vi "DT_Divide.vi"(10 "min subset size":i32=4, 11 "Points In":cluster{"x":dbl, "y":dbl, "index":i32}[](array[cluster])) -> (2 "Subset":cluster{"start idx":i32, "length":i32}[](array[cluster]), 3 "Points Out":cluster{"x":dbl, "y":dbl, "index":i32}[](array[cluster]))   [LabVIEW 2020, in "NI_AAL_Geometry.lvlib"]
uses:
  <vilib>/Analysis/NI_AAL_Geometry.lvlib
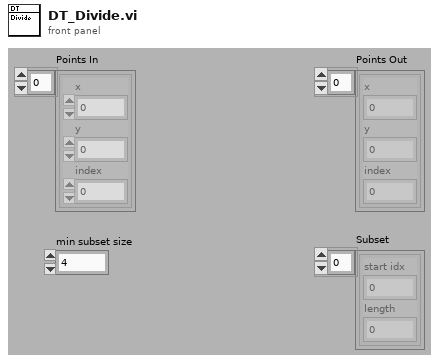
[diagram p1: front panel]
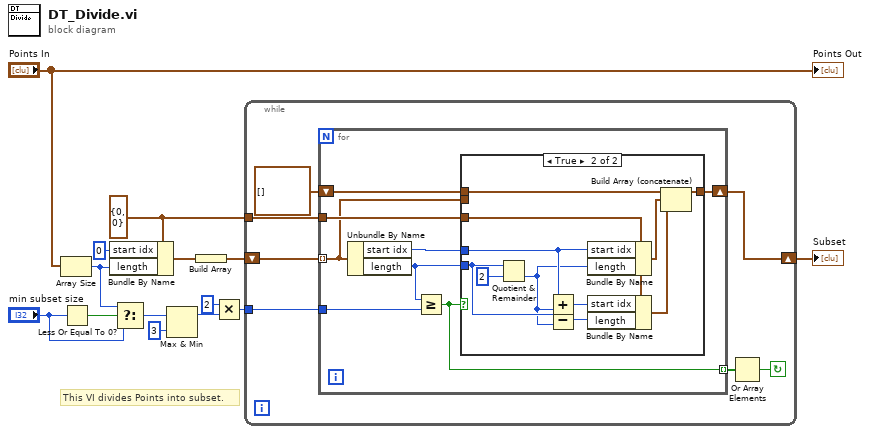
[diagram p0: block diagram]
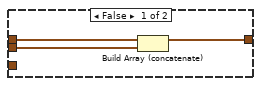
[diagram p2: hidden frame]
diagram:
  w10 = cluster{"start idx":i32, "length":i32} {"start idx"=0, "length"=0} ("subset")
  # "This VI divides Points into subset."
  n1 = Array Size(array="Points In") -> (size(s)=w6:i32)
  n2 = Less Or Equal To 0?(x="min subset size") -> (x <= 0?=w7:bool)
  n3 = Bundle By Name(cluster=w10, "start idx"=0 ("size(s)"), "length"=w6) -> (w12:cluster{"start idx":i32, "length":i32})
  n4 = Select(t=w6, s=w7, f="min subset size") -> (s? t:f=w3:i32)
  n5 = Max & Min(x=w3, y=3) -> (max(x,y)=w2:i32)  [unwired: 1 out]
  n6 = Build Array(w12) -> (w11:cluster{"start idx":i32, "length":i32}[])
  n7 = Multiply(x=2, y=w2) -> (x*y=w4:i32)
  n8 = while {
    shift-right: [w15] -> w9
    shift-left: w11 -> [w21]
    tunnel: w4 -> [w20]
    tunnel: w10 -> [w19]
    stop <- w17 continue-if-true
    n9 = for {
      tunnel: w21 -> [w22] mode=indexing
      tunnel: w20 -> [w29]
      tunnel: w19 -> [w26]
      tunnel: [w25] -> w18 mode=indexing
      shift-right: [w23] -> w15
      shift-left: cluster{"start idx":i32, "length":i32}[] [] ("Subset") -> [w24]
      n10 = Unbundle By Name(w22) -> ("start idx"=w28:i32, "length"=w27:i32)
      n11 = Greater Or Equal?(x=w27, y=w29) -> (x >= y?=w25:bool)
      n12 = case shown="True" w25 {
        tunnel: w28 -> [_ w41]
        tunnel: w27 -> [_ w34]
        tunnel: w26 -> [_ w39]
        tunnel: w24 -> [w32 w36]
        tunnel: [w30 w35] -> w23
        tunnel: w22 -> [w31 _]
        frame False {
          n13 = Build Array (concatenate)(w32, w31) -> (w30:cluster{"start idx":i32, "length":i32}[])
        }
        frame True {
          n14 = Quotient & Remainder(x=w34, y=2) -> (floor(x/y)=w33:i32)  [unwired: 1 out]
          n15 = Add(x=w41, y=w33) -> (x+y=w42:i32)
          n16 = Subtract(x=w34, y=w33) -> (x-y=w40:i32)
          n17 = Bundle By Name(cluster=w39, "start idx"=w41, "length"=w33) -> (w38:cluster{"start idx":i32, "length":i32})
          n18 = Bundle By Name(cluster=w39, "start idx"=w42, "length"=w40) -> (w37:cluster{"start idx":i32, "length":i32})
          n19 = Build Array (concatenate)(w36, w38, w37) -> (w35:cluster{"start idx":i32, "length":i32}[])
        }
      }
    }
    n20 = Or Array Elements(Boolean array=w18) -> (logical OR=w17:bool)
  }
  "Subset" <- w9
  "Points Out" <- "Points In"
